vi "Get VI ref.vi"(8 "error in (no error)":errorcluster, 10 "name":string, 11 "Control-Client in":refnum<class "Control-Client.lvclass">) -> (0 "error out":errorcluster, 2 "VI ref":refnum<vi>, 3 "Control-Client out":refnum<class "Control-Client.lvclass">)   [LabVIEW 2019, in "Control-Client.lvclass"]
uses:
  Control-Client.lvclass
  Control-Client.lvclass/Control-Client.ctl
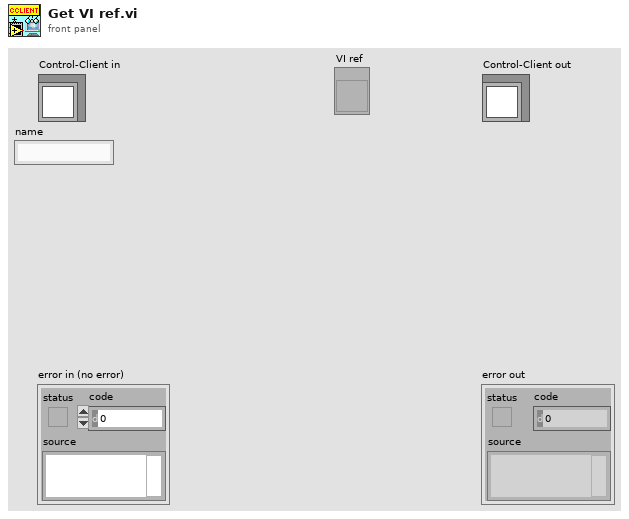
[diagram p1: front panel]
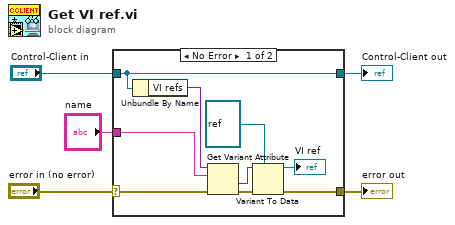
[diagram p0: block diagram]
diagram:
  n1 = case shown="No Error" "error in (no error)" {
    selector: "error in (no error)" -> [w13 w15]
    tunnel: [w11 w15] -> w4
    tunnel: [w14 w16] -> w2
    tunnel: "Control-Client in" -> [w14 w16]
    tunnel: "name" -> [w8 _]
    frame No Error {
      n2 = Unbundle By Name(w14) -> ("VI refs"=w6:variant)
      n3 = Get Variant Attribute(Variant=w6, name=w8, error in=w13) -> (value=w9:variant, error out=w12:errorcluster)  [unwired: 1 in, 2 out]
      n4 = Variant To Data(error in=w12, type=refnum<vi> refnum ("vi reference"), Variant=w9) -> (data=→"VI ref":refnum<vi>, error out=w11:errorcluster)
    }
    frame Error {
    }
  }
  "error out" <- w4
  "Control-Client out" <- w2
